vi "zad3.vi"() -> ()   [LabVIEW 2017]
panel:
  out "sorted array":dbl[][](array[numeric])
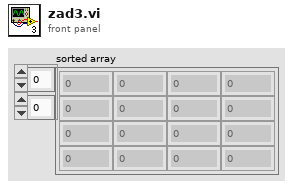
[diagram p1: front panel]
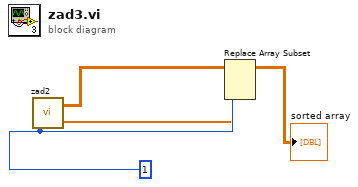
[diagram p0: block diagram]
diagram:
  w2 = 1 ("numer wiersza")
  n1 = call "zad2.vi"("numer wiersza"=w2) -> ("sorted array"=w1:dbl[], "Tablica 2d"=w3:dbl[][])  [unwired: 1 in]
  n2 = Replace Array Subset(array=w3, new element=w1, index (row)=w2) -> (→"sorted array":dbl[][])  [unwired: 1 in]
